vi "DLL-based calc.vi"() -> ()   [LabVIEW 2018]
uses:
  D:/Users_Data/Dmitriy_T/Documents/Tracker/TestVI's/Calculus.dll
  Calculus.dll
  <userlib>/_OpenG.lib/numeric/numeric.llb/Random Number Within Range - DBL__ogtk.vi
  <vilib>/Analysis/NI_AALBase.lvlib
panel:
  out "variance, us":dbl format="%0.2f"
  out "standard deviation, us":dbl format="%0.2f"
  out "mean per cycle, us":dbl format="%0.2f"
  in  "N tests":i32=10000
  out "Randoms":T1(graph)
  out "error out":errorcluster
  in  "Exit button":bool
  in  "Subtract":bool
  in  "Add":bool
  out "Result":i32
  in  "B":i32
  in  "A":i32
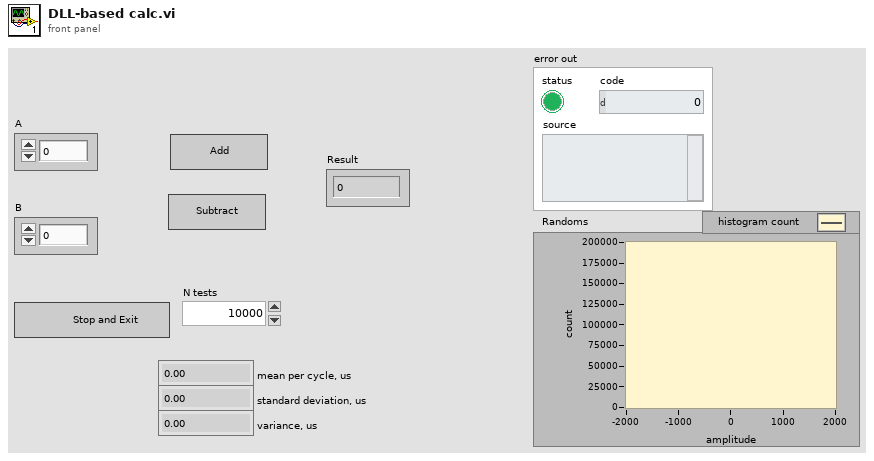
[diagram p1: front panel]
types:
  T1 = cluster{"X Values":dbl[], "Histogram: h(x)":i32[]}
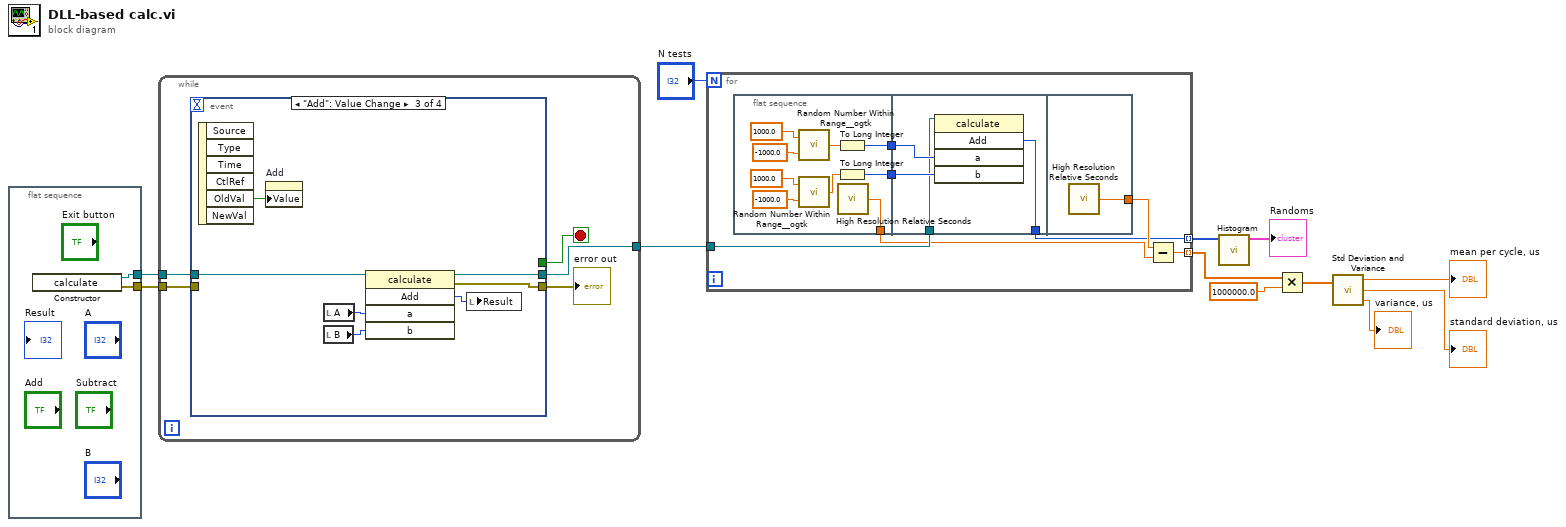
[diagram p0: block diagram]
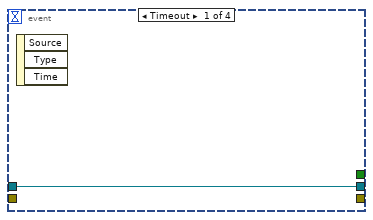
[diagram p2: hidden frame]
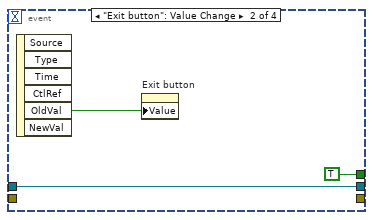
[diagram p3: hidden frame]
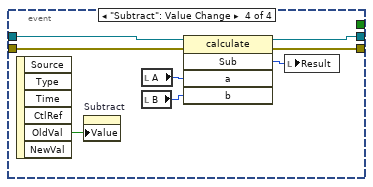
[diagram p4: hidden frame]
diagram:
  n1 = flat-sequence {
    tunnel: [w14] -> w11
    tunnel: [w13] -> w12
    frame #0 {
      n2 = constructor class="calculate"() -> (reference out=w14:refnum<k24>, error out=w13:errorcluster)  [unwired: 3 in, 1 out]
    }
  }
  n3 = while {
    tunnel: w11 -> [w18]
    tunnel: w12 -> [w17]
    tunnel: [w15] -> w10
    stop <- w19 stop-if-true
    n4 = event shown="[2] \"Add\": Value Change" {
      selector: _ -> [_ _ _ _]
      dyn-events: _ -> [_ _ _ _]
      timeout: _ -> [_ _ _ _]
      tunnel: [_ TRUE _ _] -> w19
      tunnel: w18 -> [w20 w21 w30 w38]
      tunnel: w17 -> [_ _ _ w34]
      tunnel: [_ _ w26 w33] -> w16
      tunnel: [w20 w21 w24 w31] -> w15
      event Timeout {
        n5 = event-data() -> ()  [unwired: 1 in, 3 out]
      }
      event "Exit button": Value Change {
        n6 = event-data() -> ("OldVal"=w22:bool)  [unwired: 1 in, 5 out]
        n7 = property on="Exit button" class="Bool (strict)"("Value"=w22) -> ()  [unwired: 2 in, 2 out]
      }
      event "Add": Value Change {
        n8 = event-data() -> ("OldVal"=w25:bool)  [unwired: 1 in, 5 out]
        n9 = property on="Add" class="Bool (strict)"("Value"=w25) -> ()  [unwired: 2 in, 2 out]
        n10 = local read "A"() -> (w29:i32)
        n11 = local read "B"() -> (w28:i32)
        n12 = invoke class="calculate" method="Add"(reference=w30, "a"=w29, "b"=w28) -> (reference out=w24:refnum<k24>, error out=w26:errorcluster, "Add"=w27:i32)  [unwired: 2 in, 2 out]
        n13 = local write "Result"(w27) -> ()
      }
      event "Subtract": Value Change {
        n14 = event-data() -> ("OldVal"=w32:bool)  [unwired: 1 in, 5 out]
        n15 = property on="Subtract" class="Bool (strict)"("Value"=w32) -> ()  [unwired: 2 in, 2 out]
        n16 = local read "A"() -> (w37:i32)
        n17 = local read "B"() -> (w36:i32)
        n18 = invoke class="calculate" method="Sub"(reference=w38, error in=w34, "a"=w37, "b"=w36) -> (reference out=w31:refnum<k24>, error out=w33:errorcluster, "Sub"=w35:i32)  [unwired: 1 in, 2 out]
        n19 = local write "Result"(w35) -> ()
      }
    }
    "error out" <- w16
  }
  n20 = for {
    N: "N tests" -> [_]
    tunnel: w10 -> [w43]
    tunnel: [w40] -> w8 mode=indexing
    tunnel: [w39] -> w6 mode=indexing
    n21 = flat-sequence {
      tunnel: [w49] -> w45
      tunnel: [w47] -> w44
      tunnel: [w46] -> w41
      tunnel: w45 -> [w58]
      tunnel: w44 -> [w57]
      tunnel: w43 -> [w56]
      tunnel: [w55] -> w40
      tunnel: [w59] -> w42
      frame #0 {
        n22 = call-poly <userlib>:"Random Number Within Range__ogtk.vi"("High"=1000.0, "Low"=-1000.0) -> ("Random Number"=w50:dbl)  [unwired: 3 in]
        n23 = call-poly <userlib>:"Random Number Within Range__ogtk.vi"("High"=1000.0, "Low"=-1000.0) -> ("Random Number"=w48:dbl)  [unwired: 3 in]
        n24 = To Long Integer(number=w50) -> (32bit integer=w49:i32)
        n25 = To Long Integer(number=w48) -> (32bit integer=w47:i32)
        n26 = call <vilib>:"High Resolution Relative Seconds.vi"() -> ("relative seconds"=w46:dbl)
      }
      frame #1 {
        n27 = invoke class="calculate" method="Add"(reference=w56, "a"=w58, "b"=w57) -> ("Add"=w55:i32)  [unwired: 2 in, 4 out]
      }
      frame #2 {
        n28 = call <vilib>:"High Resolution Relative Seconds.vi"() -> ("relative seconds"=w59:dbl)
      }
    }
    n29 = Subtract(x=w42, y=w41) -> (x-y=w39:dbl)
  }
  n30 = call <vilib>:"Histogram.vi"("X"=w8) -> ("Histogram Graph"=→"Randoms":T1)  [unwired: 7 in, 3 out]
  n31 = Multiply(x=w6, y=1000000.0) -> (x*y=w2:dbl[])
  n32 = call <vilib>:"Std Deviation and Variance.vi"("X"=w2) -> ("mean"=→"mean per cycle, us":dbl, "standard deviation"=→"standard deviation, us":dbl, "variance"=→"variance, us":dbl)  [unwired: 1 in]
